vi "Add Images to ImageList From ImageFiles.vi"(8 "error in (no error)":errorcluster caption="错误输入（无错误）", 10 "ImageFile Path":path[](array[path]), 11 "ImageListClass 输入":refnum<class "ImageListClass.lvclass"> caption="DNL_LabVIEW Object in") -> (0 "error out":errorcluster caption="错误输出", 3 "ImageListClass 输出":refnum<class "ImageListClass.lvclass"> caption="DNL_LabVIEW Object out")   [LabVIEW 2013, in "ImageListClass.lvclass"]
uses:
  ImageListClass.lvclass
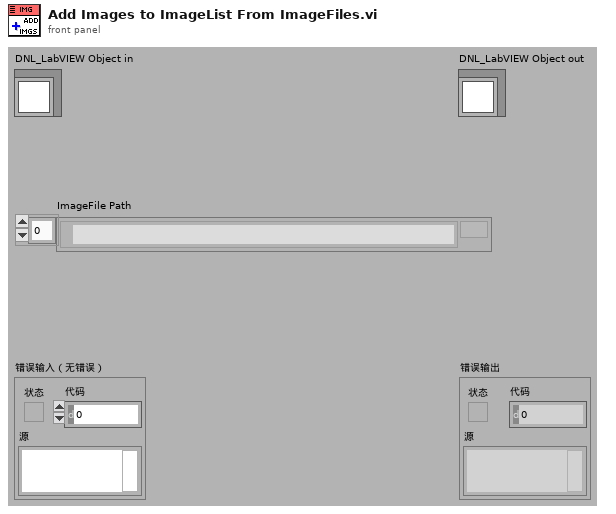
[diagram p1: front panel]
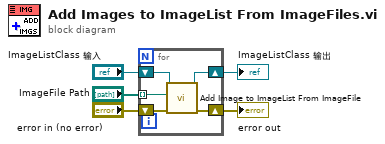
[diagram p0: block diagram]
diagram:
  n1 = for {
    shift-right: [w8] -> w4
    shift-left: "ImageListClass 输入" -> [w9]
    tunnel: "ImageFile Path" -> [w10] mode=indexing
    shift-right: [w6] -> w1
    shift-left: "error in (no error)" -> [w7]
    n2 = call "Add Image to ImageList From ImageFile.vi"("error in (no error)"=w7, "Path"=w10, "ImageListClass 输入"=w9) -> ("error out"=w6:errorcluster, "ImageListClass 输出"=w8:refnum<class "ImageListClass.lvclass">)  [unwired: 7 in]
  }
  "error out" <- w1
  "ImageListClass 输出" <- w4
